vi "pwr_sum_band.vi"(10 "df":dbl format="%.2f", 11 "In":dbl[](array[numeric]) format="%.2f") -> (3 "OUT":T1)   [LabVIEW 2013]
panel:
  out "PWR":T1(graph)
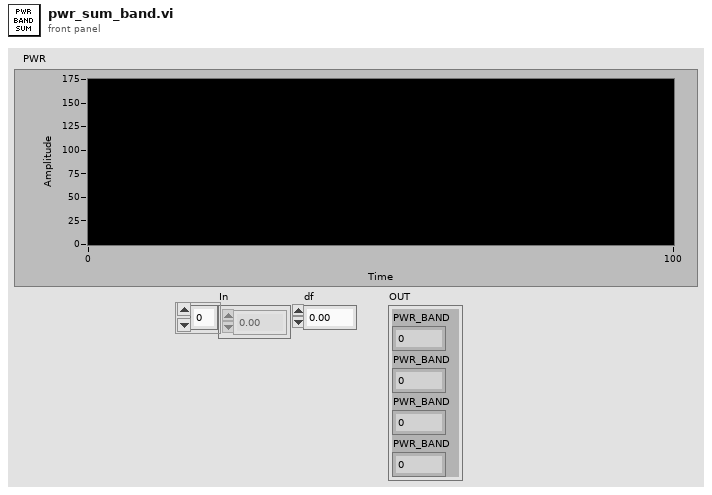
[diagram p1: front panel]
types:
  T1 = cluster{"PWR_BAND":dbl, "PWR_BAND":dbl, "PWR_BAND":dbl, "PWR_BAND":dbl}
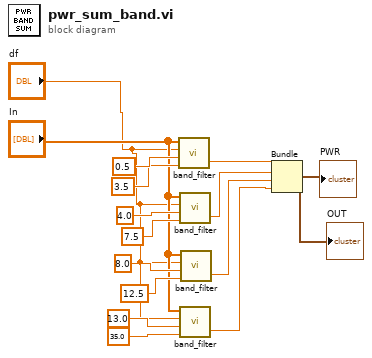
[diagram p0: block diagram]
diagram:
  n1 = call "band_filter.vi"("hi_freq"=3.5, "low_Freq"=0.5, "df"="df", "In"="In") -> ("PWR_BAND"=w13:dbl)  [unwired: 1 out]
  n2 = call "band_filter.vi"("hi_freq"=7.5, "low_Freq"=4.0, "df"="df", "In"="In") -> ("PWR_BAND"=w10:dbl)  [unwired: 1 out]
  n3 = call "band_filter.vi"("hi_freq"=35.0, "low_Freq"=13.0, "df"="df", "In"="In") -> ("PWR_BAND"=w4:dbl)  [unwired: 1 out]
  n4 = call "band_filter.vi"("hi_freq"=12.5, "low_Freq"=8.0, "df"="df", "In"="In") -> ("PWR_BAND"=w7:dbl)  [unwired: 1 out]
  n5 = Bundle("PWR_BAND"=w13, "PWR_BAND"=w10, "PWR_BAND"=w7, "PWR_BAND"=w4) -> (→"PWR" →"OUT":T1)  [unwired: 1 in]
